vi "MGI Monitored Actor.vi"   [LabVIEW 2017]
uses:
  <vilib>/Platform/browser.llb/Open URL in Default Browser (string).vi
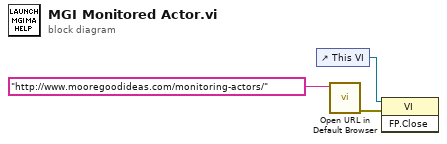
[diagram p0: block diagram]
diagram:
  n1 = control-ref of="This VI"() -> (w1:refnum<vi>)
  n2 = call-poly <vilib>:"Open URL in Default Browser.vi"("URL"="http://www.mooregoodideas.com/monitoring-actors/") -> ("error out"=w2:errorcluster)  [unwired: 5 in, 1 out]
  n3 = invoke class="VI" method="FP.Close"(reference=w1, error in=w2) -> ()  [unwired: 1 in, 3 out]
